vi "GetDataFlowTimestamp.vi"(11 "data":T1) -> (2 "unix timestamp":i64, 3 "has waveforms":bool)   [LabVIEW 2017, in "DataEventCreator.lvlib"]
uses:
  <vilib>/addons/InsightCM/Devices/Shared/Common/DataEventCreator/DataEventCreator.lvlib
  <vilib>/addons/InsightCM/Devices/Shared/Common/DataFlow/controls/Data.ctl
  <vilib>/addons/InsightCM/Utilities/DataAccessors/controls/wfmSGL_DVR.ctl
  <vilib>/addons/PointValueMap/controls/PointMap.ctl
  <vilib>/addons/InsightCM/Devices/Shared/Common/DataFlow/controls/Type.ctl
  <vilib>/addons/PointValueMap/PointValueMap.lvlib
  <vilib>/addons/InsightCM/Devices/Shared/Common/DataFlow/DataFlow.lvlib
panel:
  out "timestamp":timestamp
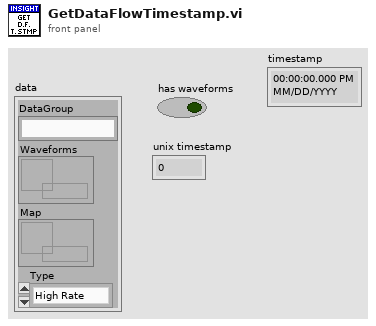
[diagram p1: front panel]
types:
  T1 = typedef "DataFlow.lvlib/Data.ctl" = cluster{"DataGroup":string, "Waveforms":T2, "Map":T3, "Type":T4}
  T2 = typedef "wfmSGL_DVR.ctl" = refnum<data-value>
  T3 = typedef "PointValueMap.lvlib/PointMap.ctl" = refnum<data-value>
  T4 = typedef "DataFlow.lvlib/Type.ctl" = enum16{"High Rate", "Low Rate", "Burst Mode"}
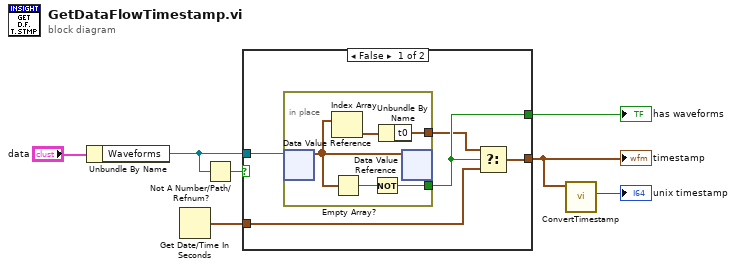
[diagram p0: block diagram]
diagram:
  n1 = Unbundle By Name("data") -> ("Waveforms"=w6:T2)
  n2 = Get Date/Time In Seconds() -> (seconds since 1Jan1904=w3:timestamp)
  n3 = Not A Number/Path/Refnum?(number/path/refnum=w6) -> (NaN/Path/Refnum?=w1:bool)
  n4 = case shown="False" w1 {
    tunnel: [w9 w18] -> w4
    tunnel: w6 -> [w12 _]
    tunnel: [w11 _] -> w7
    tunnel: w3 -> [w10 w18]
    frame False {
      n5 = in-place {
        in-place-border: [w16] -> w8
        in-place-border: [w13] -> w11
        n6 = in-place-dvr #1(w12) -> (w15:waveform(sgl)[])  [unwired: 1 out]
        n7 = Index Array(array=w15) -> (element=w17:waveform(sgl))  [unwired: 1 in]
        n8 = Empty Array?(array=w15) -> (empty?=w14:bool)
        n9 = Not(x=w14) -> (.not. x?=w13:bool)
        n10 = Unbundle By Name(w17) -> ("t0"=w16:timestamp)
        n11 = in-place-dvr #1(w15) -> ()  [unwired: 2 out]
      }
      n12 = Select(t=w8, s=w11, f=w10) -> (s? t:f=w9:timestamp)
    }
    frame True {
    }
  }
  "has waveforms" <- w7
  "timestamp" <- w4
  n13 = call <vilib>:"ConvertTimestamp.vi"("Time Stamp"=w4) -> ("Timestamp out"=→"unix timestamp":i64)  [unwired: 10 in]
